vi "Read Prep.vi"(8 "error in (no error)":errorcluster, 11 "Readable in":refnum<class "Readable.lvclass">) -> (0 "error out":errorcluster, 3 "Readable out":refnum<class "Readable.lvclass">)   [LabVIEW 2012, in "Readable.lvclass"]
doc: "(Dynamic) Prepare to read. This is in case the Readable object needs to change some settings before the time delay occurs. One example: if the photon counter needs to start counting, call this method and then wait until the count is complete. The \"_Read\" method will then stop counting and return the total counts."
uses:
  Readable.lvclass
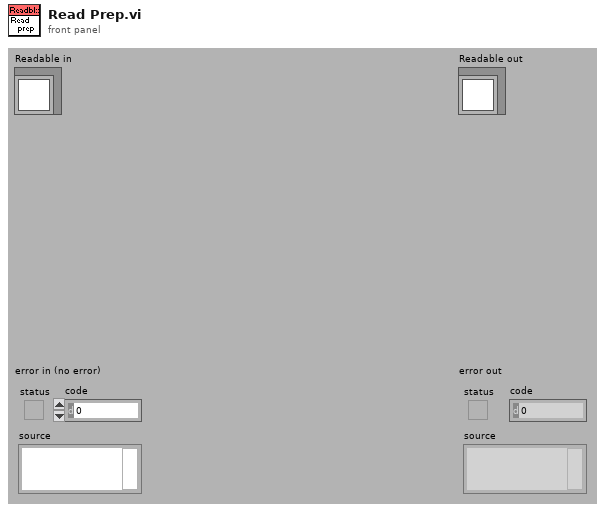
[diagram p1: front panel]
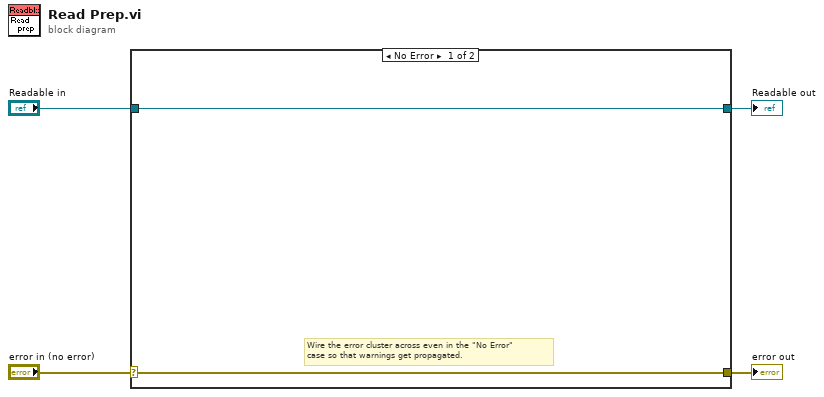
[diagram p0: block diagram]
diagram:
  n1 = case shown="No Error" "error in (no error)" {
    selector: "error in (no error)" -> [w5 w8]
    tunnel: [w5 w8] -> w3
    tunnel: [w6 w7] -> w1
    tunnel: "Readable in" -> [w6 w7]
    frame No Error {
      # "Wire the error cluster across even in the \"No Error\"\ncase so that warnings get propagated."
    }
    frame Error {
    }
  }
  "error out" <- w3
  "Readable out" <- w1
